vi "initialize.vi"(0 "NInstrSim_ConfigureVDCRange":refnum<class "NInstrSim_ConfigureVDCRange.lvclass">, 3 "initializationData":variant, 5 "error in (no error)":errorcluster, 7 "binaryString":string, 8 "I8 Array":i8[](array[numeric]), 9 "prependSize? (T)":bool, 11 "byteOrder (0:big-endian, network order)":T1(ring)) -> (14 "dup NInstrSim_ConfigureVDCRange":refnum<class "NInstrSim_ConfigureVDCRange.lvclass">, 17 "found?":bool, 19 "error out":errorcluster)   [LabVIEW 2009, in "HB_Device_Examples.lvlib" / "NInstrSim_ConfigureVDCRange.lvclass"]
doc: "This is a dynamic dispatch VI to be implemented by child classes to initialize their attributes.\n\n<B>Recommendation:</B> Use Variant for initialization data."
uses:
  NInstrSim_ConfigureVDCRange.lvclass
  NInstrSim_Visitor.lvclass
  NInstrSim_ConfigureVDCRange.lvclass/NInstrSim_ConfigureVDCRange.ctl
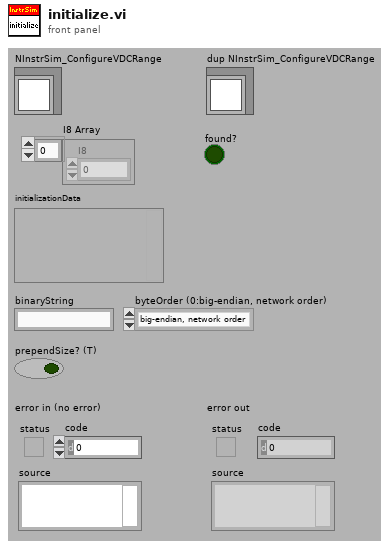
[diagram p1: front panel]
types:
  T1 = enum16{"big-endian, network order", "native, host order", "little-endian"}
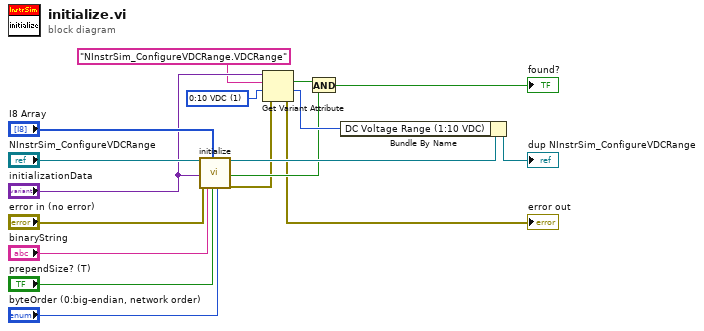
[diagram p0: block diagram]
diagram:
  w10 = u16 1 items=["0:1 VDC", "0:10 VDC", "0:100 VDC"] ("DC Voltage Range (1:10 VDC)")
  n1 = call-parent "initialize.vi"("HGF_NetworkData"="NInstrSim_ConfigureVDCRange", "initializationData"="initializationData", "error in (no error)"="error in (no error)", "binaryString"="binaryString", "I8 Array"="I8 Array", "prependSize? (T)"="prependSize? (T)", "byteOrder (0:big-endian, network order)"="byteOrder (0:big-endian, network order)") -> ("dup HGF_NetworkData"=w8:refnum<class "NInstrSim_ConfigureVDCRange.lvclass">, "found?"=w4:bool, "error out"=w2:errorcluster)  [unwired: 10 out]
  n2 = Get Variant Attribute(Variant="initializationData", name="NInstrSim_ConfigureVDCRange.VDCRange", default value (empty Variant)=w10, error in=w2) -> (found=w5:bool, value=w6:u16, error out=→"error out":errorcluster)  [unwired: 1 out]
  n3 = And(x=w5, y=w4) -> (x .and. y?=→"found?":bool)
  n4 = Bundle By Name(cluster=w8, "DC Voltage Range (1:10 VDC)"=w6) -> (→"dup NInstrSim_ConfigureVDCRange":refnum<class "NInstrSim_ConfigureVDCRange.lvclass">)
